vi "Build Directory File.vi"() -> ()   [LabVIEW 2013]
uses:
  <vilib>/Utility/file.llb/Write To Spreadsheet File (string).vi
panel:
  out "#":i32
  out "filenames":string[](array[string])
  in  "path":path
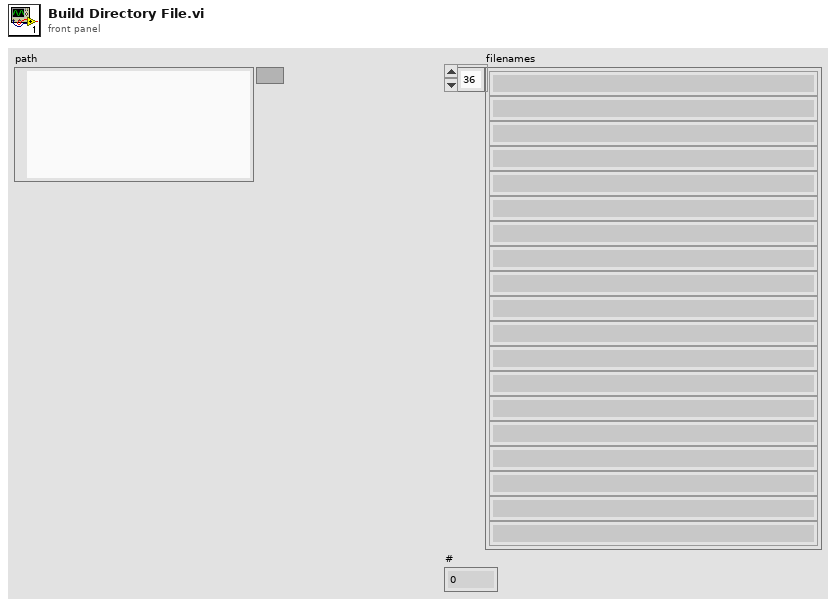
[diagram p1: front panel]
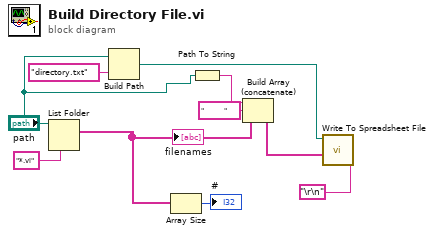
[diagram p0: block diagram]
diagram:
  n1 = List Folder(path="path", pattern="*.vi") -> (filenames=w5:string[])  [unwired: 2 in, 3 out]
  "filenames" <- w5
  n2 = Build Path(base path="path", name or relative path="directory.txt") -> (appended path=w6:path)
  n3 = Array Size(array=w5) -> (size(s)=→"#":i32)
  n4 = Path To String(path="path") -> (string=w4:string)
  n5 = Build Array (concatenate)(w4, "          " ("element"), w5) -> (w2:string[])
  n6 = call-poly <vilib>:"Write To Spreadsheet File.vi"("delimiter (\\t)"="\r\n", "1D data"=w2, "file path (dialog if empty)"=w6) -> ()  [unwired: 5 in, 1 out]
